vi "Get Cycle Count.vi"(8 "error in (no error)":errorcluster, 10 "Clear?":bool) -> (0 "error out":errorcluster, 1 "timed out?":bool, 2 "Reply Payload":T1)   [LabVIEW 2015, in "Tool Module.lvlib"]
doc: "Get the cycle count value. If Clear is set TRUE then clear the cycle count to 0 in the tool.\n_____\nCreated using Delacor QMH Event Scripter 3.1.0.29."
uses:
  Tool Module.lvlib
  Get Cycle Count (Reply Payload)--cluster.ctl
  Get Cycle Count Argument--cluster.ctl
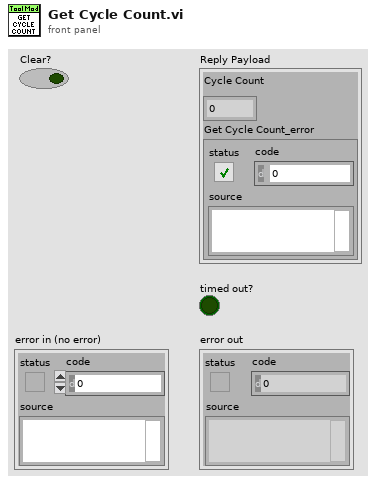
[diagram p1: front panel]
types:
  T1 = typedef "Tool Module.lvlib/Get Cycle Count (Reply Payload)--cluster.ctl" = cluster{"Cycle Count":i32, "Get Cycle Count_error":errorcluster}
  T2 = typedef "Tool Module.lvlib/Get Cycle Count Argument--cluster.ctl" = cluster{"Clear?":bool, "Wait Notifier":refnum<notifier>}
  T3 = typedef "Tool Module.lvlib/Request Events--cluster.ctl" = cluster{"Stop Module":refnum<user-event>, "Show Panel":refnum<user-event>, "Hide Panel":refnum<user-event>, "Get Module Execution Status":refnum<user-event>, "Show Diagram":refnum<user-event>, "Test Trig 2":refnum<user-event>, "GOTO":refnum<user-event>, "Start Inspect":refnum<user-event>, "CONNECT":refnum<user-event>, "Get All Inspect Data":refnum<user-event>, "Get Inspection Limits":refnum<user-event>, "Set Inspection Limits":refnum<user-event>, "Update Status":refnum<user-event>, "Start Data Monitor":refnum<user-event>, "Get FPGA Setup Params":refnum<user-event>, "Set FPGA Setup Params":refnum<user-event>, "Set Tool Config":refnum<user-event>, "Get Tool Config":refnum<user-event>, "Set Integration Count":refnum<user-event>, "Set Laser Params":refnum<user-event>, "Get Mtrl Ctrl Reg":refnum<user-event>, "Commit Ctrl Reg":refnum<user-event>, "Set Event Logger":refnum<user-event>, "Write to File":refnum<user-event>, "Read from File":refnum<user-event>, "Set Device Temp Thresholds":refnum<user-event>, "Get Cycle Count":refnum<user-event>}
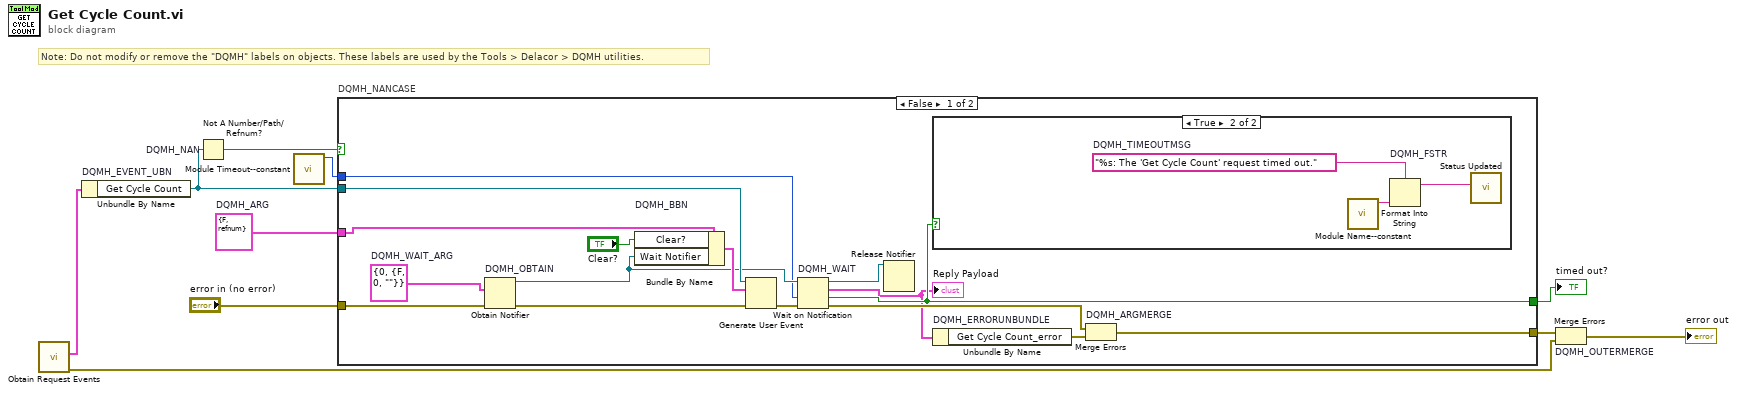
[diagram p0: block diagram]
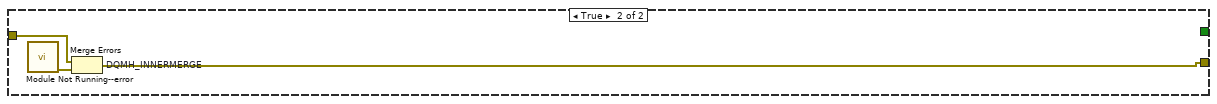
[diagram p3: hidden frame]
diagram:
  w4 = T2 {"Clear?"=FALSE, "Wait Notifier"=refnum}  # DQMH_ARG
  # "Note: Do not modify or remove the \"DQMH\" labels on objects. These labels are used by the Tools > Delacor > DQMH utilities."
  n1 = call "Obtain Request Events.vi"() -> ("error out"=w2:errorcluster, "Tool Module Request Events"=w1:T3)  [unwired: 10 in]
  n2 = Unbundle By Name "DQMH_EVENT_UBN"(w1) -> ("Get Cycle Count"=w8:refnum<user-event>)
  n3 = Not A Number/Path/Refnum? "DQMH_NAN"(number/path/refnum=w8) -> (NaN/Path/Refnum?=w7:bool)
  n4 = call "Module Timeout--constant.vi"() -> ("Module Timeout"=w3:i32)  [unwired: 11 in]
  n5 = case "DQMH_NANCASE" shown="False" w7 {
    tunnel: "error in (no error)" -> [w26 w32]
    tunnel: w8 -> [w24 _]
    tunnel: [w16 w31] -> w5
    tunnel: [w17 _] -> w6
    tunnel: w4 -> [w13 _]
    tunnel: w3 -> [w11 _]
    frame False {
      w21 = T1 {"Cycle Count"=0, "Get Cycle Count_error"={"status"=FALSE, "code"=0, "source"=""}}  # DQMH_WAIT_ARG
      n6 = Obtain Notifier "DQMH_OBTAIN"(notification data type=w21, error in (no error)=w26) -> (notifier out=w19:refnum<notifier>, error out=w22:errorcluster)  [unwired: 2 in, 1 out]
      n7 = Bundle By Name "DQMH_BBN"(cluster=w13, "Clear?"="Clear?", "Wait Notifier"=w19) -> (w23:T2)
      n8 = Generate User Event(user event=w24, event data cluster=w23, error in=w22) -> (error out=w25:errorcluster)  [unwired: 1 in, 1 out]
      n9 = Wait on Notification "DQMH_WAIT"(notifier=w19, timeout in ms (-1)=w11, error in (no error)=w25) -> (notifier out=w18:refnum<notifier>, notification=w14:T1, timed out?=w17:bool, error out=w20:errorcluster)  [unwired: 1 in]
      "Reply Payload" <- w14
      n10 = Release Notifier(notifier=w18) -> ()  [unwired: 2 in, 3 out]
      n11 = case shown="True" w17 {
        frame False {
        }
        frame True {
          w29 = "%s: The 'Get Cycle Count' request timed out."  # DQMH_TIMEOUTMSG
          n12 = call "Module Name--constant.vi"() -> ("Module Name"=w28:string)  [unwired: 11 in]
          n13 = Format Into String "DQMH_FSTR"(format string=w29, w28) -> (resulting string=w27:string)  [unwired: 2 in, 1 out]
          n14 = call "Status Updated.vi"("Status"=w27) -> ()  [unwired: 10 in, 1 out]
        }
      }
      n15 = Unbundle By Name "DQMH_ERRORUNBUNDLE"(w14) -> ("Get Cycle Count_error"=w15:errorcluster)
      n16 = Merge Errors "DQMH_ARGMERGE"(w20, w15) -> (w16:errorcluster)
    }
    frame True {
      n17 = call "Module Not Running--error.vi"() -> ("error out"=w30:errorcluster)  [unwired: 11 in]
      n18 = Merge Errors "DQMH_INNERMERGE"(w32, w30) -> (w31:errorcluster)
    }
  }
  "timed out?" <- w6
  n19 = Merge Errors "DQMH_OUTERMERGE"(w5, w2) -> (→"error out":errorcluster)
